vi "DequeueEventLogger.vi"(8 "error in (no error)":errorcluster, 11 "Queue in":refnum<queue>) -> (0 "error out":errorcluster, 1 "Data":variant, 2 "Message":T1, 3 "Queue out":refnum<queue>)   [LabVIEW 2019, in "EventLogger.lvlib"]
uses:
  EventLogger.lvlib
  Enum - Message.ctl
  Cluster - MessageCluster.ctl
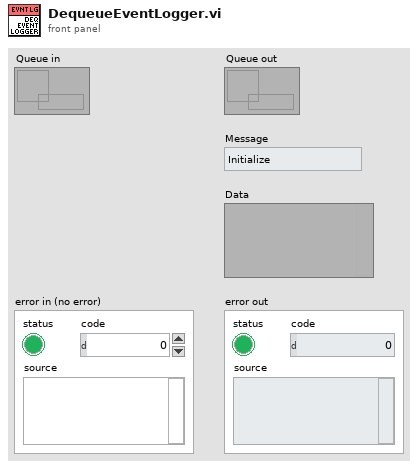
[diagram p1: front panel]
types:
  T1 = typedef "EventLogger.lvlib/Enum - Message.ctl" = enum16{"Initialize", "Idle", "CreateLog", "LogStrEvent", "LogErrorEvent", "LogVICall", "Error", "Exit"}
  T2 = typedef "EventLogger.lvlib/Cluster - MessageCluster.ctl" = cluster{"Message":T1, "Data":variant}
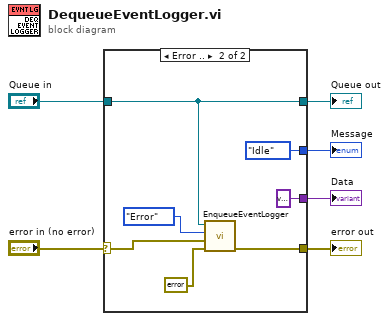
[diagram p0: block diagram]
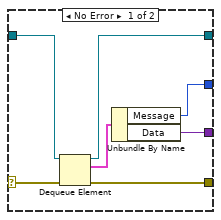
[diagram p2: hidden frame]
diagram:
  n1 = case shown="Error .." "error in (no error)" {
    selector: "error in (no error)" -> [w7 w17]
    tunnel: [w13 variant ("Data")] -> w6
    tunnel: [w12 Enum_-_Message."Idle" ("Message")] -> w5
    tunnel: "Queue in" -> [w10 w19]
    tunnel: [w9 w19] -> w3
    tunnel: [w8 w20] -> w2
    frame No Error {
      n2 = Dequeue Element(queue=w10, error in (no error)=w7) -> (queue out=w9:refnum<queue>, element=w11:T2, error out=w8:errorcluster)  [unwired: 1 in, 1 out]
      n3 = Unbundle By Name(w11) -> ("Message"=w12:T1, "Data"=w13:variant)
    }
    frame Error {
      n4 = call "EnqueueEventLogger.vi"("Error In"=errorcluster {"status"=FALSE, "code"=0, "source"=""}, "Data"=w17, "Message"=Enum_-_Message."Error", "EventLoggerQueue"=w19) -> ("Error Out"=w20:errorcluster)  [unwired: 6 in, 1 out]
    }
  }
  "Data" <- w6
  "Message" <- w5
  "Queue out" <- w3
  "error out" <- w2
